vi "ExX2CamerasSameGraph.vi"() -> ()   [LabVIEW 2010]
panel:
  out "Camera 16":sgl[](graph)
  out "Camera 15":sgl[](graph)
  out "Camera 14":sgl[](graph)
  out "Camera 13":sgl[](graph)
  out "Camera 12":sgl[](graph)
  out "Camera 11":sgl[](graph)
  out "Camera 10":sgl[](graph)
  out "Camera 9":sgl[](graph)
  out "Camera 8":sgl[](graph)
  out "Camera 7":sgl[](graph)
  out "Camera 6":sgl[](graph)
  out "Camera 5":sgl[](graph)
  out "Camera 4":sgl[](graph)
  out "Camera 3":sgl[](graph)
  out "Camera 2":sgl[](graph)
  out "Camera 1":sgl[](graph)
  in  "stop":bool
  in  "Exposure":dbl=0.5 format="%.2f"
  out "error out":errorcluster
  in  "error in (no error)":errorcluster
  # "Ex2CamerasSameGraph:\nThis example runs two cameras in focus mode.\nSets them up for center strip and displays as graph.\nRemember to setup two cameras in the pvcam.ini\nfile."
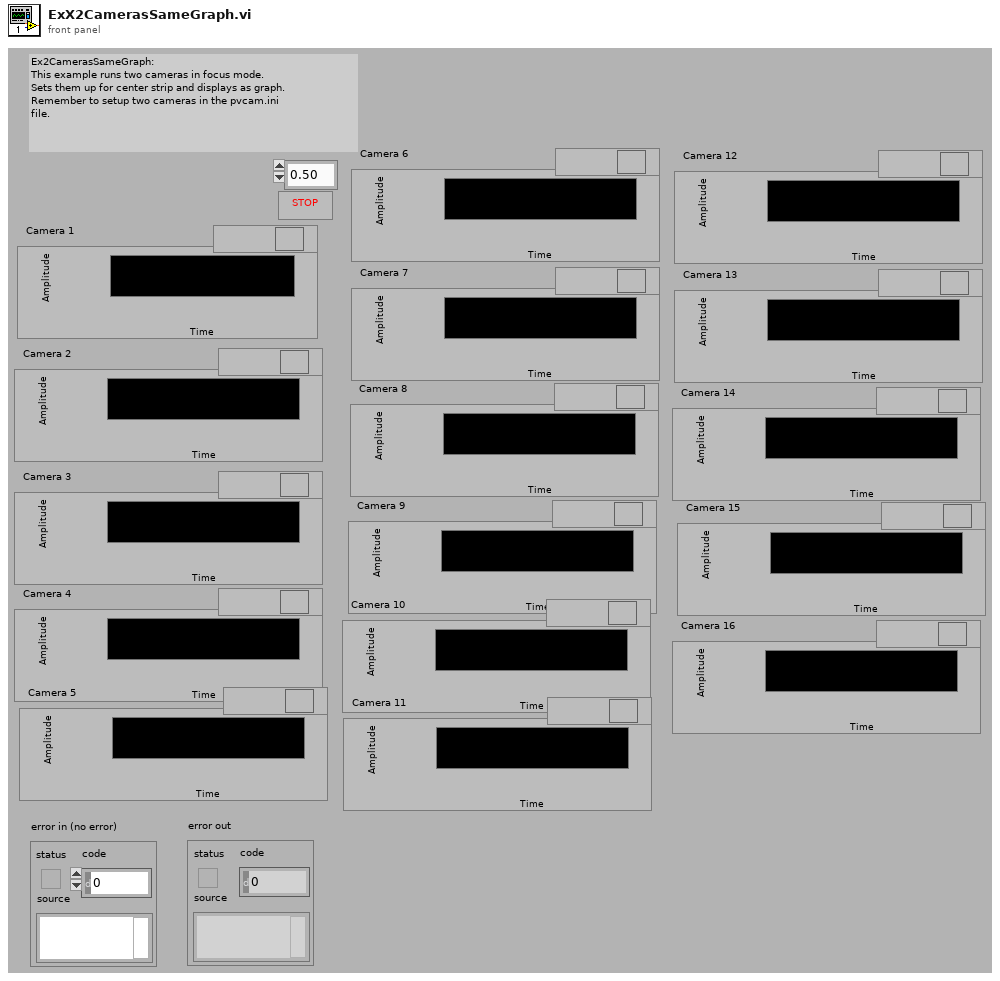
[diagram p1: front panel]
types:
  T1 = cluster{"Camera Handle":u32, "Camera Handle":u32}
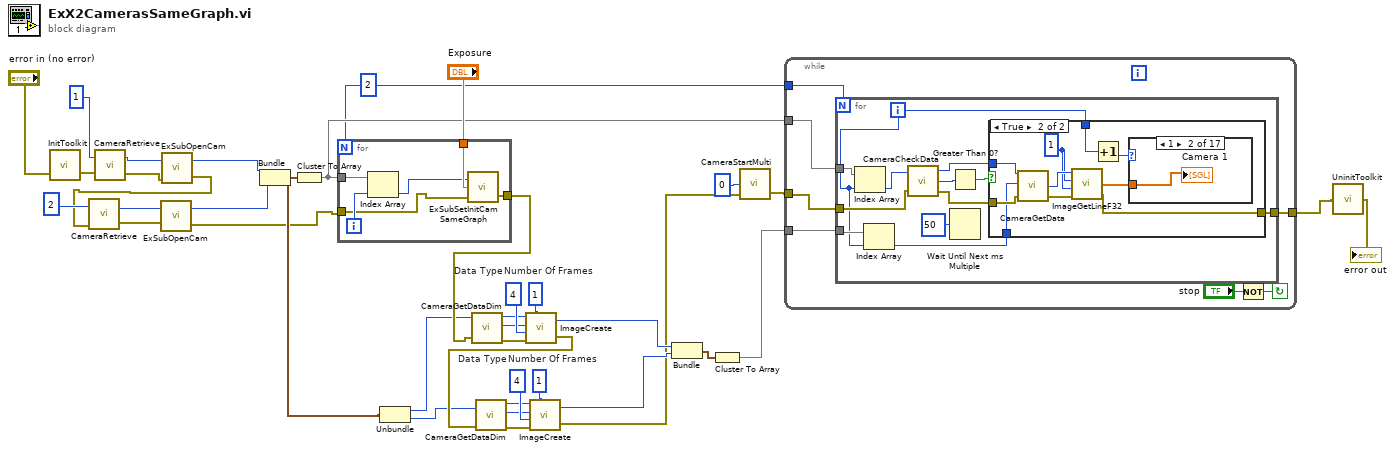
[diagram p0: block diagram]
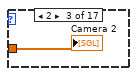
[diagram p4: hidden frame]
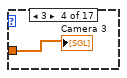
[diagram p5: hidden frame]
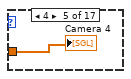
[diagram p6: hidden frame]
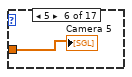
[diagram p7: hidden frame]
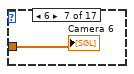
[diagram p8: hidden frame]
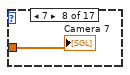
[diagram p9: hidden frame]
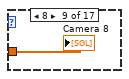
[diagram p10: hidden frame]
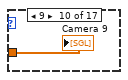
[diagram p11: hidden frame]
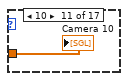
[diagram p12: hidden frame]
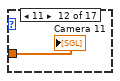
[diagram p13: hidden frame]
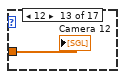
[diagram p14: hidden frame]
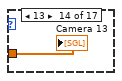
[diagram p15: hidden frame]
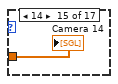
[diagram p16: hidden frame]
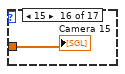
[diagram p17: hidden frame]
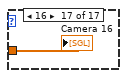
[diagram p18: hidden frame]
diagram:
  w21 = u32 1  # Number Of Frames
  w22 = u32 4  # Data Type
  w26 = u32 1  # Number Of Frames
  w27 = u32 4  # Data Type
  w29 = 2
  n1 = call <userlib>:"InitToolkit.vi"("error in"="error in (no error)") -> ("error out"=w38:errorcluster)
  n2 = call <userlib>:"CameraRetrieve.vi"("error in"=w38, "Camera Index"=1) -> ("error out"=w5:errorcluster, "Device ID"=w8:u32)
  n3 = call "ExSubOpenCam.vi"("error in (no error)"=w5, "Camera Device ID"=w8) -> ("error out"=w4:errorcluster, "Camera Handle"=w7:u32)
  n4 = call <userlib>:"CameraRetrieve.vi"("error in"=w4, "Camera Index"=2) -> ("error out"=w3:errorcluster, "Device ID"=w1:u32)
  n5 = call "ExSubOpenCam.vi"("error in (no error)"=w3, "Camera Device ID"=w1) -> ("error out"=w2:errorcluster, "Camera Handle"=w6:u32)
  n6 = Bundle("Camera Handle"=w7, "Camera Handle"=w6) -> (w10:T1)  [unwired: 1 in]
  n7 = Cluster To Array(cluster=w10) -> (array=w32:u32[])
  n8 = for {
    N: w29 -> [_]
    tunnel: w32 -> [w45]
    tunnel: [w43] -> w15
    tunnel: "Exposure" -> [w42]
    tunnel: w2 -> [w41]
    i -> [w44]
    n9 = Index Array(array=w45, index=w44) -> (element=w40:u32)
    n10 = call "ExSubSetInitCamSameGraph.vi"("error in (no error)"=w41, "Exposure"=w42, "Camera Handle"=w40) -> ("error out"=w43:errorcluster)  [unwired: 1 out]
  }
  n11 = Unbundle(w10) -> ("Camera Handle"=w13:u32, "Camera Handle"=w12:u32)
  n12 = call <userlib>:"CameraGetDataDim.vi"("Camera Handle"=w13, "error in"=w15) -> ("Xdim"=w24:u32, "Ydim"=w25:u32, "error out"=w28:errorcluster)  [unwired: 1 out]
  n13 = call <userlib>:"ImageCreate.vi"("X dimension"=w24, "Y dimension"=w25, "Data Type"=w27, "error in"=w28, "Number Of Frames"=w26) -> ("Image Handle"=w18:u32, "error out"=w14:errorcluster)
  n14 = call <userlib>:"CameraGetDataDim.vi"("Camera Handle"=w12, "error in"=w14) -> ("Xdim"=w19:u32, "Ydim"=w20:u32, "error out"=w23:errorcluster)  [unwired: 1 out]
  n15 = call <userlib>:"ImageCreate.vi"("X dimension"=w19, "Y dimension"=w20, "Data Type"=w22, "error in"=w23, "Number Of Frames"=w21) -> ("Image Handle"=w17:u32, "error out"=w9:errorcluster)
  n16 = Bundle("Image Handle"=w18, "Image Handle"=w17) -> (w11:cluster{"Image Handle":u32, "Image Handle":u32})  [unwired: 1 in]
  n17 = Cluster To Array(cluster=w11) -> (array=w16:u32[])
  n18 = call "CameraStartMulti.vi"("error in (no error)"=w9, "Number Of Cameras"=0) -> ("error out"=w34:errorcluster)  [unwired: 1 in, 1 out]
  n19 = while {
    tunnel: w34 -> [w49]
    tunnel: w32 -> [w50]
    tunnel: [w48] -> w30
    tunnel: w29 -> [w47]
    tunnel: w16 -> [w46]
    stop <- w51 continue-if-true
    n20 = for {
      N: w47 -> [_]
      tunnel: [w59] -> w48
      tunnel: w50 -> [w58]
      tunnel: w49 -> [w56]
      tunnel: w46 -> [w55]
      i -> [w53]
      n21 = Index Array(array=w58, index=w53) -> (element=w57:u32)
      n22 = Index Array(array=w55, index=w53) -> (element=w54:u32)
      n23 = call <userlib>:"CameraCheckData.vi"("Camera Handle"=w57, "error in"=w56) -> ("Camera Handle"=w61:u32, "Number Of Frames Available"=w63:i32, "error out"=w60:errorcluster)
      n24 = Greater Than 0?(x=w63) -> (x > 0?=w62:bool)
      n25 = Wait Until Next ms Multiple(millisecond multiple=u32 50) -> ()  [unwired: 1 out]
      n26 = case shown="True" w62 {
        tunnel: [w65 w72] -> w59
        tunnel: w61 -> [_ w71]
        tunnel: w60 -> [w65 w70]
        tunnel: w53 -> [_ w66]
        tunnel: w54 -> [_ w68]
        frame False {
        }
        frame True {
          w73 = 1
          n27 = call <userlib>:"CameraGetData.vi"("error in"=w70, "Data Handle"=w68, "Camera Handle"=w71) -> ("error out"=w75:errorcluster, "Data Handle"=w74:u32)  [unwired: 1 out]
          n28 = call <userlib>:"ImageGetLineF32.vi"("error in"=w75, "Z Position"=w73, "Y Position"=w73, "Data Handle"=w74) -> ("error out"=w72:errorcluster, "Array F32"=w69:sgl[])  [unwired: 1 out]
          n29 = Increment(x=w66) -> (x+1=w67:i32)
          n30 = case shown="1" w67 {
            tunnel: w69 -> [_ w76 w77 w78 w79 w80 w81 w82 w83 w84 w85 w86 w87 w88 w89 w90 w91]
            frame Default {
            }
            frame 1 {
              "Camera 1" <- w76
            }
            frame 2 {
              "Camera 2" <- w77
            }
            frame 3 {
              "Camera 3" <- w78
            }
            frame 4 {
              "Camera 4" <- w79
            }
            frame 5 {
              "Camera 5" <- w80
            }
            frame 6 {
              "Camera 6" <- w81
            }
            frame 7 {
              "Camera 7" <- w82
            }
            frame 8 {
              "Camera 8" <- w83
            }
            frame 9 {
              "Camera 9" <- w84
            }
            frame 10 {
              "Camera 10" <- w85
            }
            frame 11 {
              "Camera 11" <- w86
            }
            frame 12 {
              "Camera 12" <- w87
            }
            frame 13 {
              "Camera 13" <- w88
            }
            frame 14 {
              "Camera 14" <- w89
            }
            frame 15 {
              "Camera 15" <- w90
            }
            frame 16 {
              "Camera 16" <- w91
            }
          }
        }
      }
    }
    n31 = Not(x="stop") -> (.not. x?=w51:bool)
  }
  n32 = call <userlib>:"UninitToolkit.vi"("error in"=w30) -> ("error out"=→"error out":errorcluster)
